vi "GetText.vi"(8 "error in":errorcluster, 11 "StepNode in":refnum<class "StepNode.lvclass">) -> (0 "error out":errorcluster, 1 "additional text":string, 2 "text":string, 3 "StepNode Out":refnum<class "StepNode.lvclass">, 4 "glyph":string)   [LabVIEW 2015, in "StepNode.lvclass"]
doc: "Copyright 2017 National Instruments Corporation\n\nLicensed under the Apache License, Version 2.0 (the \"License\"); you may not use this file except in compliance with the License. You may obtain a copy of the License at http://www.apache.org/licenses/LICENSE-2.0\nUnless required by applicable law or agreed to in writing, software distributed under the License is distributed on an \"AS IS\" BASIS, WITHOUT WARRANTIES OR CONDITIONS OF ANY KIND, either express or implied. See the License for the specific language governing permissions and limitations under the License."
uses:
  StepNode.lvclass
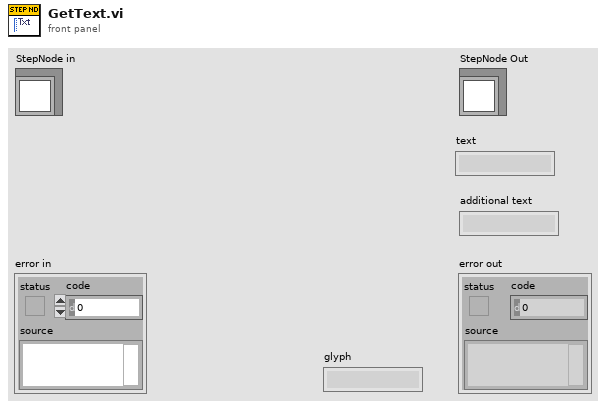
[diagram p1: front panel]
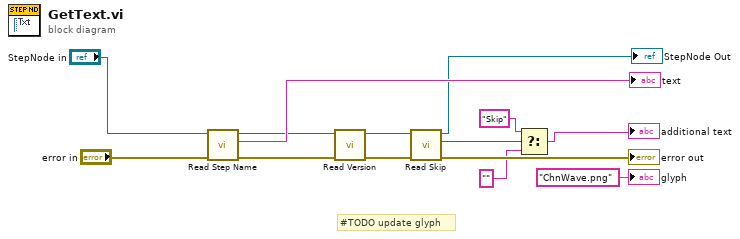
[diagram p0: block diagram]
diagram:
  # "#TODO update glyph"
  n1 = call-dynamic "Read Step Name.vi"("error in (no error)"="error in", "StepNode in"="StepNode in") -> ("error out"=w7:errorcluster, "Step Name"=→"text":string, "StepNode out"=w4:refnum<class "StepNode.lvclass">)  [unwired: 7 in]
  n2 = call-dynamic "Read Version.vi"("error in (no error)"=w7, "StepNode in"=w4) -> ("error out"=w8:errorcluster, "StepNode out"=w3:refnum<class "StepNode.lvclass">)  [unwired: 7 in, 1 out]
  n3 = call-dynamic "Read Skip.vi"("error in (no error)"=w8, "StepNode in"=w3) -> ("error out"=→"error out":errorcluster, "Skip"=w11:bool, "StepNode out"=→"StepNode Out":refnum<class "StepNode.lvclass">)  [unwired: 7 in]
  n4 = Select(t="Skip", s=w11, f="") -> (s? t:f=→"additional text":string)
  "glyph" <- "ChnWave.png" ("glyph")
